vi "Read header.vi"(8 "error in (no error)":errorcluster, 11 "JSONWebToken in":refnum<class "JSONWebToken.lvclass">) -> (0 "error out":errorcluster, 2 "JWT header":T1, 3 "JSONWebToken out":refnum<class "JSONWebToken.lvclass">)   [LabVIEW 2024]
uses:
  JSONWebToken.lvclass
  header.ctl
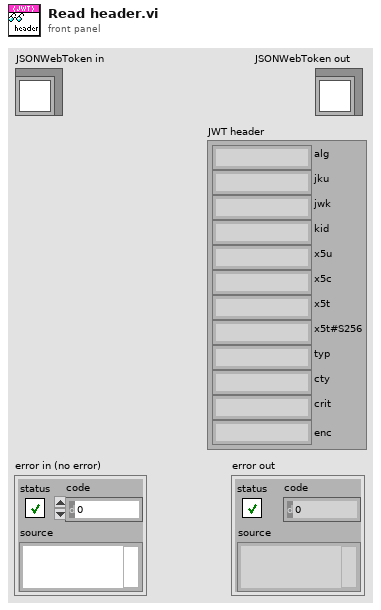
[diagram p1: front panel]
types:
  T1 = typedef "header.ctl" = cluster{"alg":string, "jku":string, "jwk":string, "kid":string, "x5u":string, "x5c":string, "x5t":string, "x5t#S256":string, "typ":string, "cty":string, "crit":string, "enc":string}
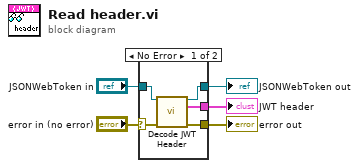
[diagram p0: block diagram]
diagram:
  n1 = case shown="No Error" "error in (no error)" {
    selector: "error in (no error)" -> [w7 w11]
    tunnel: [w6 w11] -> w4
    tunnel: [w9 w12] -> w2
    tunnel: "JSONWebToken in" -> [w10 w12]
    tunnel: [w8 _] -> w1
    frame No Error {
      n2 = call "Decode JWT Header.vi"("JSONWebToken in"=w10, "error in (no error)"=w7) -> ("JSONWebToken out"=w9:refnum<class "JSONWebToken.lvclass">, "JWT header"=w8:T1, "error out"=w6:errorcluster)  [unwired: 10 in, 1 out]
    }
    frame Error {
    }
  }
  "error out" <- w4
  "JSONWebToken out" <- w2
  "JWT header" <- w1
